vi "CRYMR_TOL2.vi"(0 "Tolerance":u16(ring)=1 items=["Individual Points", "Absolute Limits", "Floating Limits", "Floating Data", "Aligned Limits", "Aligned Data"], 1 "X Floating Limits":u16(ring) items=["No", "Yes"], 2 "x axis":enum32{"Linear", "Log"}(ring), 5 "Limits":u16(ring)=2 items=["Upper Only", "Lower Only", "Upper & Lower"], 6 "X min-max-step":T1={"Limit X Offset Min"=0.0, "Limit X Offset Max"=500.0, "Limit X Offset Step Size"=10.0} {"Limit X Offset Step Size" step=0.01 format="%.2f"; "Limit X Offset Max" step=0.01 format="%.2f"; "Limit X Offset Min" step=0.01 format="%.2f"}, 7 "Data":cluster{"Hz":dbl, "dB":dbl}[](array[cluster])=[{"Hz"=200.0, "dB"=2.9}, {"Hz"=500.0, "dB"=3.5}, {"Hz"=1000.0, "dB"=5.0}, {"Hz"=2000.0, "dB"=6.0}, {"Hz"=4500.0, "dB"=4.0}] {"dB" format="%.1f"}, 9 "Upper Limit":cluster{"Hz":dbl, "y":dbl}[](array[cluster])=[{"Hz"=300.0, "y"=4.0}, {"Hz"=1000.0, "y"=6.5}, {"Hz"=4000.0, "y"=5.0}, {"Hz"=5000.0, "y"=4.2}] {"y" format="%.1f"}, 11 "Lower Limit":cluster{"Hz":dbl, "y":dbl}[](array[cluster])=[{"Hz"=400.0, "y"=0.5}, {"Hz"=1000.0, "y"=3.5}, {"Hz"=3000.0, "y"=1.5}] {"y" format="%.1f"}, 12 "Align Reference":cluster{dbl, dbl}={1250.0, 4.5} {"?" format="%.1f"}, 13 "Resolution (decimals)":i32=2) -> (3 "Margin":dbl=-0.25 format="%.1f", 4 "Verdict":bool, 8 "Data Out":cluster{dbl, dbl}[](array[cluster])=[{200.00000000000003, 2.9}, {499.99999999999994, 3.5}, {1000.0, 5.0}, {2000.0000000000002, 6.0}, {4499.999999999998, 4.0}] {"?" format="%.2f"; "?" format="%.2f"}, 10 "Upper Limit Out":cluster{dbl, dbl}[](array[cluster])=[{300.0000000000001, 4.0}, {1000.0, 6.5}, {4000.000000000001, 5.0}, {4999.999999999999, 4.2}] {"?" format="%.2f"; "?" format="%.2f"}, 14 "Align Reference Out":cluster{dbl, dbl}={1250.0, 4.5} {"?" format="%.1f"}, 15 "Lower Limit Out":cluster{dbl, dbl}[](array[cluster])=[{400.0000000000001, 0.5}, {1000.0, 3.5}, {3000.000000000001, 1.5}] {"?" format="%.2f"; "?" format="%.2f"})   [LabVIEW 2013]
uses:
  CRYLimit edit global.vi
panel:
  out "Lo Fail":cluster{dbl, dbl}[](array[cluster])
  out "Up Fail":cluster{dbl, dbl}[](array[cluster])
  out "verdict out":bool
  out "align ref point":cluster{dbl, dbl}[](array[cluster])
  out "Align Ref":cluster{dbl, dbl}
  out "Critical":cluster{dbl, dbl}[](array[cluster])
  out "Margin out":dbl
  out "Data output":cluster{dbl, dbl}[](array[cluster])
  out "Low out":cluster{dbl, dbl}[](array[cluster])
  out "Up out":cluster{dbl, dbl}[](array[cluster])
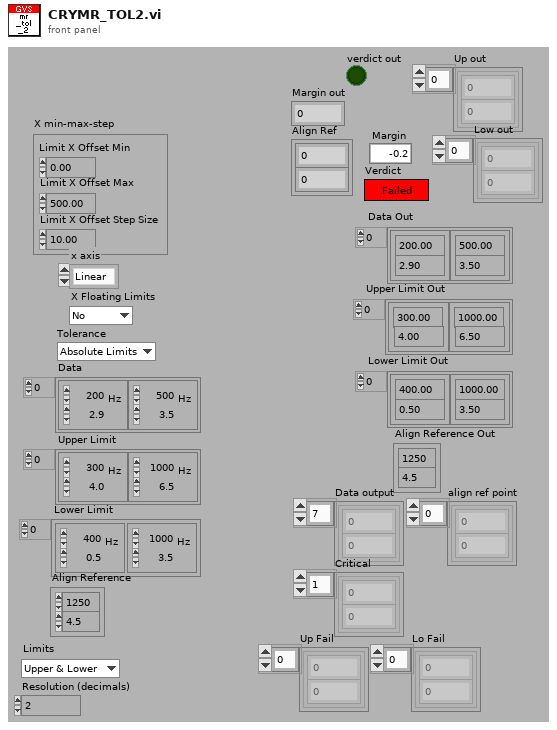
[diagram p1: front panel]
types:
  T1 = cluster{"Limit X Offset Min":dbl, "Limit X Offset Max":dbl, "Limit X Offset Step Size":dbl}
  T2 = cluster{"Data X Offset":dbl, "Data Y Offset":dbl}
  T3 = cluster{"Limit X Offset Min":dbl, "Limit Y Offset":dbl}
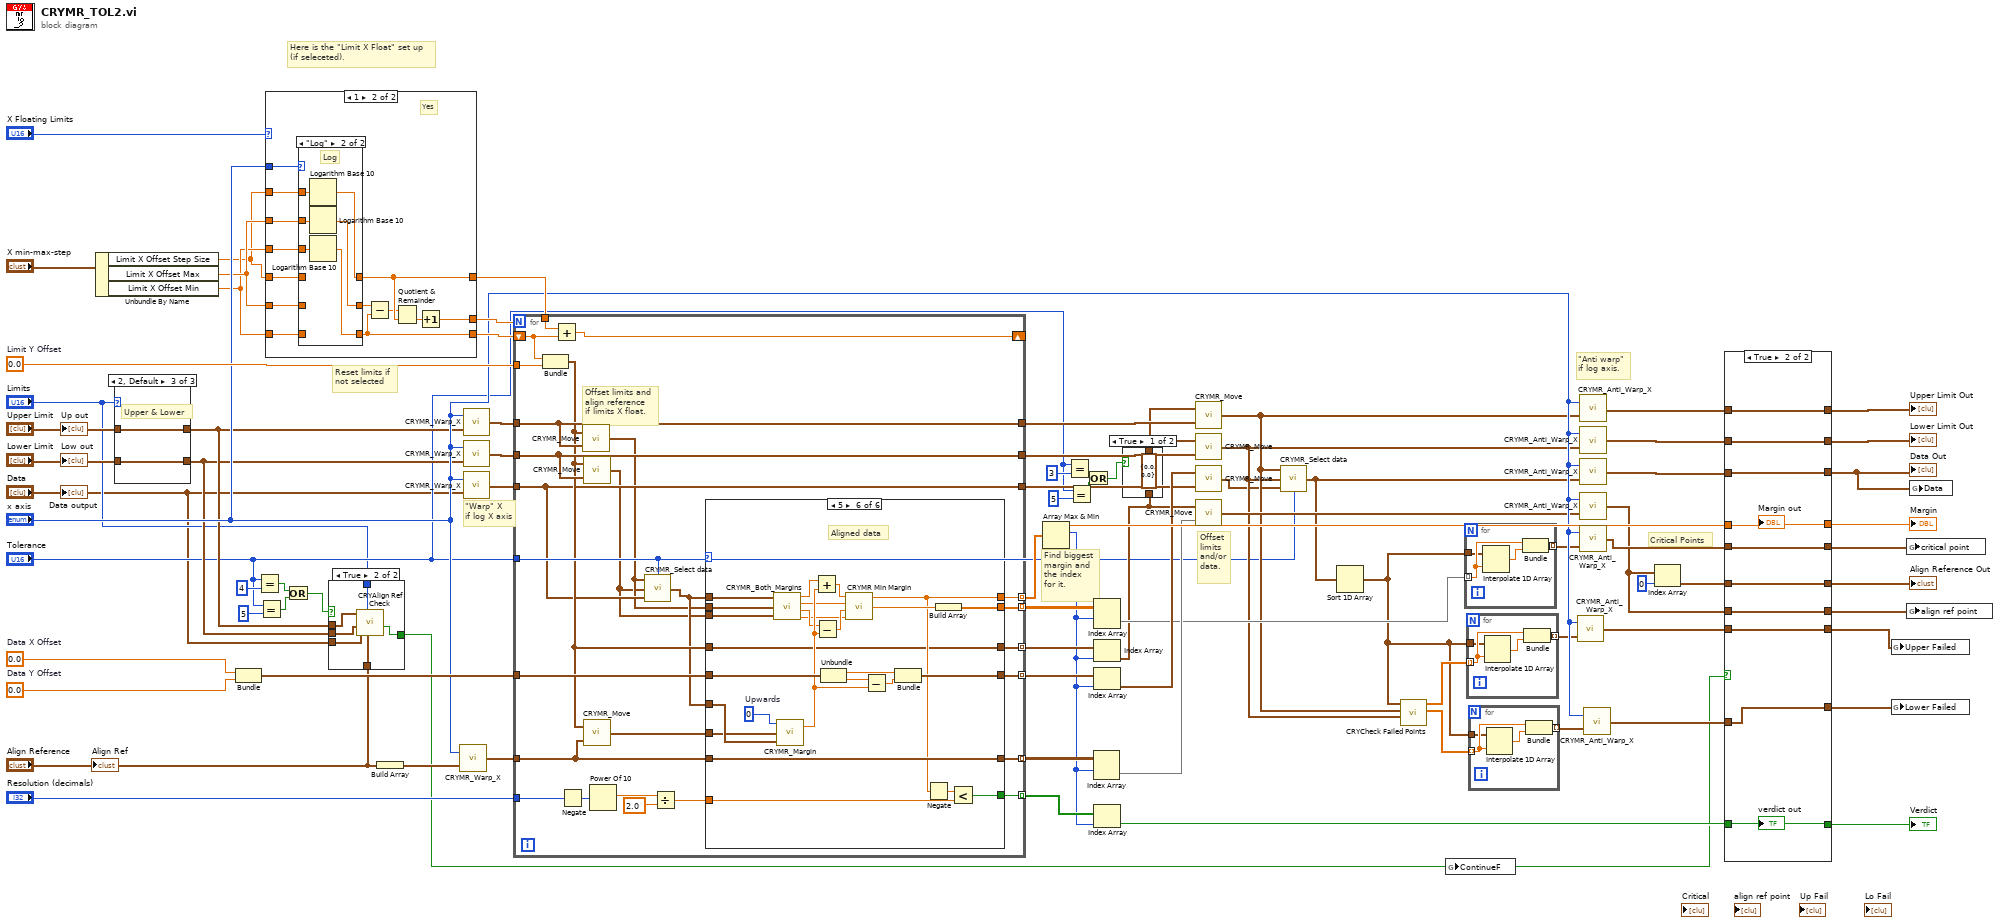
[diagram p0: block diagram]
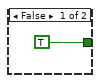
[diagram p3: hidden frame]
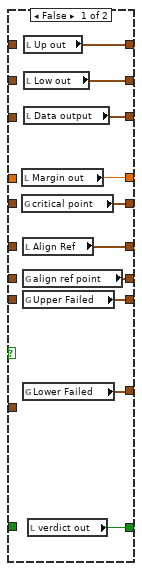
[diagram p4: hidden frame]
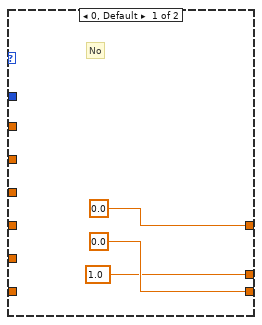
[diagram p5: hidden frame]
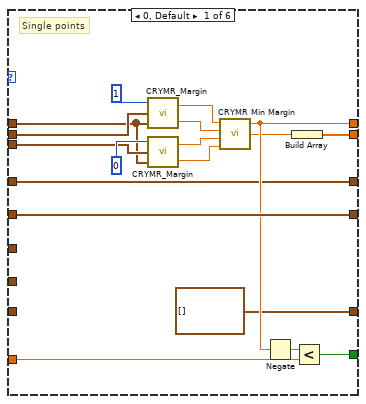
[diagram p7: hidden frame]
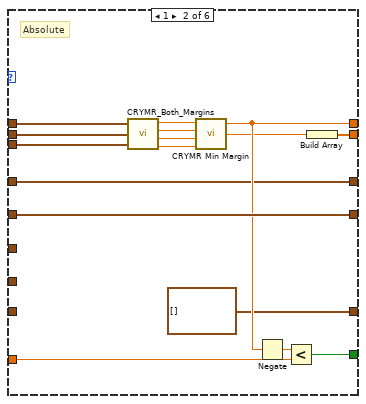
[diagram p8: hidden frame]
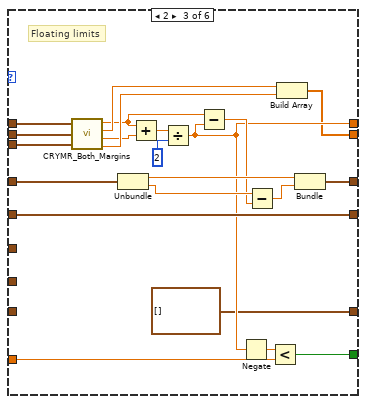
[diagram p9: hidden frame]
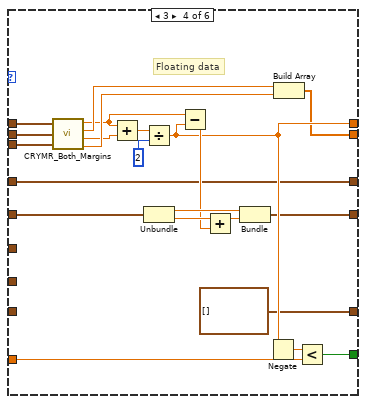
[diagram p10: hidden frame]
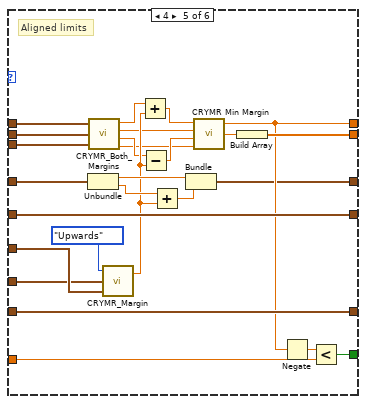
[diagram p11: hidden frame]
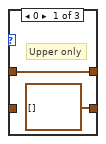
[diagram p12: hidden frame]
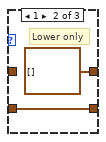
[diagram p13: hidden frame]
diagram:
  w56 = 0.0  # Data Y Offset
  w57 = 0.0  # Data X Offset
  w61 = 0.0  # Limit Y Offset
  # "\"Anti warp\"\nif log axis."
  # "Critical Points"
  # "Find biggest\nmargin and \nthe index\nfor it."
  # "Offset \nlimits\nand/or\ndata."
  # "\"Warp\" X \nif log X axis"
  # "Reset limits if \nnot selected"
  # "Here is the \"Limit X Float\" set up\n(if seleceted)."
  n1 = Unbundle By Name("X min-max-step") -> ("Limit X Offset Step Size"=w38:dbl, "Limit X Offset Max"=w40:dbl, "Limit X Offset Min"=w39:dbl)
  n2 = case shown="2, Default" "Limits" {
    tunnel: "Upper Limit" -> [w87 _ w91]
    tunnel: [w87 cluster{"Hz":dbl, "y":dbl}[] [] ("Upper Limit") w91] -> w29
    tunnel: "Lower Limit" -> [_ w89 w90]
    tunnel: [cluster{"Hz":dbl, "y":dbl}[] [] ("Lower Limit") w89 w90] -> w28
    frame 0 {
      # "Upper only"
    }
    frame 1 {
      # "Lower only"
    }
    frame 2, Default {
      # "Upper & Lower"
    }
  }
  n3 = Bundle("Data X Offset"=w57, "Data Y Offset"=w56) -> (w52:T2)  [unwired: 1 out]
  n4 = Equal?(x="Tolerance", y=u16 4) -> (x = y?=w17:bool)
  n5 = Equal?(x="Tolerance", y=u16 5) -> (x = y?=w16:bool)
  n6 = case shown="1" "X Floating Limits" {
    tunnel: w38 -> [_ w101]
    tunnel: w40 -> [_ w103]
    tunnel: w39 -> [_ w106]
    tunnel: w39 -> [_ w104]
    tunnel: [0.0 w102] -> w43
    tunnel: w40 -> [_ w105]
    tunnel: [0.0 w100] -> w45
    tunnel: [1.0 w98] -> w44
    tunnel: "x axis" -> [_ w107]
    tunnel: w38 -> [_ w99]
    frame 0, Default {
      # "No"
    }
    frame 1 {
      # "Yes"
      n7 = case shown="\"Log\"" w107 {
        tunnel: w106 -> [_ w116]
        tunnel: w105 -> [w110 _]
        tunnel: [w110 w113] -> w97
        tunnel: w104 -> [w109 _]
        tunnel: [w109 w114] -> w102
        tunnel: w103 -> [_ w115]
        tunnel: w101 -> [w108 _]
        tunnel: [w108 w111] -> w100
        tunnel: w99 -> [_ w112]
        frame "Linear", Default {
          # "Lin"
        }
        frame "Log" {
          # "Log"
          n8 = Logarithm Base 10(1:w112) -> (0:w111:dbl)
          n9 = Logarithm Base 10(1:w115) -> (0:w113:dbl)
          n10 = Logarithm Base 10(1:w116) -> (0:w114:dbl)
        }
      }
      n11 = Subtract(x=w97, y=w102) -> (x-y=w96:dbl)
      n12 = Quotient & Remainder(x=w96, y=w100) -> (floor(x/y)=w95:dbl)  [unwired: 1 out]
      n13 = Increment(x=w95) -> (x+1=w98:dbl)
    }
  }
  n14 = Or(x=w17, y=w16) -> (x .or. y?=w3:bool)
  n15 = case shown="True" w3 {
    tunnel: w29 -> [_ w123]
    tunnel: w28 -> [_ w122]
    tunnel: "Align Reference" -> [_ w121]
    tunnel: [TRUE ("Align Flag") w118] -> w12
    tunnel: "Limits" -> [_ w120]
    tunnel: "Data" -> [_ w119]
    frame False {
    }
    frame True {
      n16 = call "CRYAlign Ref Check.vi"("Align Reference"=w121, "Limits"=w120, "Data"=w119, "Lower Limit"=w122, "Upper Limit"=w123) -> ("Align Flag"=w118:bool)  [unwired: 6 in]
    }
  }
  n17 = Build Array("Align Reference") -> (w51:cluster{dbl, dbl}[])
  n18 = call "CRYMR_Warp_X.vi"("Input"=w51, "x axis"="x axis") -> ("Output"=w50:cluster{dbl, dbl}[])
  n19 = call "CRYMR_Warp_X.vi"("Input"=w29, "x axis"="x axis") -> ("Output"=w53:cluster{dbl, dbl}[])
  n20 = call "CRYMR_Warp_X.vi"("Input"=w28, "x axis"="x axis") -> ("Output"=w54:cluster{dbl, dbl}[])
  n21 = call "CRYMR_Warp_X.vi"("Input"="Data", "x axis"="x axis") -> ("Output"=w49:cluster{dbl, dbl}[])
  n22 = for {
    N: w44 -> [_]
    tunnel: "Resolution (decimals)" -> [w129]
    tunnel: "Tolerance" -> [w124]
    tunnel: w54 -> [w134]
    tunnel: w53 -> [w135]
    tunnel: [w128] -> w64
    tunnel: [w134] -> w63
    tunnel: [w135] -> w62
    tunnel: [w144] -> w47 mode=indexing
    tunnel: [w143] -> w66 mode=indexing
    tunnel: [w142] -> w67 mode=indexing
    tunnel: [w141] -> w68 mode=indexing
    tunnel: w61 -> [w131]
    tunnel: [w140] -> w60 mode=indexing
    tunnel: w50 -> [w133]
    shift-right: [w138] -> _
    shift-left: w43 -> [w132]
    tunnel: [w137] -> w58 mode=indexing
    tunnel: w49 -> [w128]
    tunnel: w45 -> [w136]
    tunnel: w52 -> [w145]
    # "Offset limits and\nalign reference\nif limits X float."
    n23 = Bundle("Limit X Offset Min"=w132, "Limit Y Offset"=w131) -> (w130:T3)  [unwired: 1 out]
    n24 = Add(x=w136, y=w132) -> (x+y=w138:dbl)
    n25 = Negate(x=w129) -> (-x=w147:i32)
    n26 = call "CRYMR_Move.vi"("Input"=w135, "Offsets"=w130) -> ("Output"=w126:cluster{dbl, dbl}[])
    n27 = call "CRYMR_Move.vi"("Input"=w134, "Offsets"=w130) -> ("Output"=w125:cluster{dbl, dbl}[])
    n28 = call "CRYMR_Move.vi"("Input"=w133, "Offsets"=w130) -> ("Output"=w139:cluster{dbl, dbl}[])
    n29 = Power Of 10(x=w147) -> (10^x=w146:dbl)
    n30 = call "CRYMR_Select data.vi"("Tolerance"=w124, "Data"=w128, "Lower Limit"=w125, "Upper Limit"=w126) -> ("Data Out"=w127:cluster{dbl, dbl}[])
    n31 = Divide(x=w146, y=2.0) -> (x/y=w149:dbl)
    n32 = case shown="5" w124 {
      tunnel: [w166 w182 w201 w223 w252 w277] -> w141
      tunnel: w149 -> [w165 w181 w202 w224 w253 w278]
      tunnel: w127 -> [w150 w168 w186 w208 w244 w257]
      tunnel: w126 -> [w156 w170 w185 w207 w243 w256]
      tunnel: w125 -> [w155 w169 w184 w206 w242 w255]
      tunnel: w145 -> [w164 w180 w200 w209 w251 w269]
      tunnel: [w164 w180 w200 w217 w251 w268] -> w142
      tunnel: [w159 w172 w195 w210 w228 w254] -> w143
      tunnel: [w163 w179 w194 w218 w246 w258] -> w144
      tunnel: [w162 w177 w193 w216 w249 w265] -> w140
      tunnel: w127 -> [_ _ _ _ w250 w274]
      tunnel: w139 -> [_ _ _ _ w248 w264]
      tunnel: [cluster{dbl, dbl}[] [] cluster{dbl, dbl}[] [] cluster{dbl, dbl}[] [] cluster{dbl, dbl}[] [] w247 w263] -> w137
      tunnel: w133 -> [_ _ _ _ w247 w263]
      tunnel: w130 -> [w159 w172 w187 w210 w245 w254]
      frame 0, Default {
        # "Single points"
        n33 = call "CRYMR_Margin.vi"("To"=w150, "From"=w156, "Direction"=1) -> ("X"=w153:dbl, "Margin"=w154:dbl)
        n34 = call "CRYMR_Margin.vi"("To"=w150, "From"=w155, "Direction"=0) -> ("X"=w151:dbl, "Margin"=w152:dbl)
        n35 = call "CRYMR Min Margin.vi"("Lower X"=w151, "Lower Margin"=w152, "Upper X"=w153, "Upper Margin"=w154) -> ("X"=w161:dbl, "Min Margin"=w163:dbl)  [unwired: 1 out]
        n36 = Negate(x=w163) -> (-x=w167:dbl)
        n37 = Build Array(w161) -> (w162:dbl[])
        n38 = Less?(x=w167, y=w165) -> (x < y?=w166:bool)
      }
      frame 1 {
        # "Absolute"
        n39 = call "CRYMR_Both_Margins.vi"("Data"=w168, "Upper Limit"=w170, "Lower Limit"=w169) -> ("Upper Margin"=w171:dbl, "Upper Margin X"=w173:dbl, "Lower Margin"=w174:dbl, "Lower Margin X"=w175:dbl)
        n40 = call "CRYMR Min Margin.vi"("Lower X"=w175, "Lower Margin"=w174, "Upper X"=w173, "Upper Margin"=w171) -> ("X"=w178:dbl, "Min Margin"=w179:dbl)  [unwired: 1 out]
        n41 = Negate(x=w179) -> (-x=w183:dbl)
        n42 = Less?(x=w183, y=w181) -> (x < y?=w182:bool)
        n43 = Build Array(w178) -> (w177:dbl[])
      }
      frame 2 {
        # "Floating limits"
        n44 = call "CRYMR_Both_Margins.vi"("Data"=w186, "Upper Limit"=w185, "Lower Limit"=w184) -> ("Upper Margin"=w189:dbl, "Upper Margin X"=w190:dbl, "Lower Margin"=w188:dbl, "Lower Margin X"=w191:dbl)
        n45 = Unbundle(w187) -> ("Limit X Offset Min"=w199:dbl, "Limit Y Offset"=w198:dbl)
        n46 = Add(x=w189, y=w188) -> (x+y=w205:dbl)
        n47 = Divide(x=w205, y=2) -> (x/y=w194:dbl)
        n48 = Subtract(x=w189, y=w194) -> (x-y=w196:dbl)
        n49 = Negate(x=w194) -> (-x=w203:dbl)
        n50 = Subtract(x=w198, y=w196) -> (x-y=w197:dbl)
        n51 = Less?(x=w203, y=w202) -> (x < y?=w201:bool)
        n52 = Build Array(w190, w191) -> (w193:dbl[])
        n53 = Bundle("Limit X Offset Min"=w199, w197) -> (w195:cluster{"Limit X Offset Min":dbl, dbl})  [unwired: 1 out]
      }
      frame 3 {
        # "Floating data"
        n54 = call "CRYMR_Both_Margins.vi"("Data"=w208, "Upper Limit"=w207, "Lower Limit"=w206) -> ("Upper Margin"=w212:dbl, "Upper Margin X"=w213:dbl, "Lower Margin"=w211:dbl, "Lower Margin X"=w214:dbl)
        n55 = Add(x=w212, y=w211) -> (x+y=w227:dbl)
        n56 = Divide(x=w227, y=2) -> (x/y=w218:dbl)
        n57 = Unbundle(w209) -> ("Data X Offset"=w222:dbl, "Data Y Offset"=w221:dbl)
        n58 = Subtract(x=w212, y=w218) -> (x-y=w219:dbl)
        n59 = Add(x=w221, y=w219) -> (x+y=w220:dbl)
        n60 = Bundle("Data X Offset"=w222, w220) -> (w217:cluster{"Data X Offset":dbl, dbl})  [unwired: 1 out]
        n61 = Negate(x=w218) -> (-x=w225:dbl)
        n62 = Build Array(w213, w214) -> (w216:dbl[])
        n63 = Less?(x=w225, y=w224) -> (x < y?=w223:bool)
      }
      frame 4 {
        # "Aligned limits"
        n64 = Unbundle(w245) -> ("Limit X Offset Min"=w240:dbl, "Limit Y Offset"=w239:dbl)
        n65 = call "CRYMR_Both_Margins.vi"("Data"=w244, "Upper Limit"=w243, "Lower Limit"=w242) -> ("Upper Margin"=w233:dbl, "Upper Margin X"=w232:dbl, "Lower Margin"=w231:dbl, "Lower Margin X"=w230:dbl)
        n66 = call "CRYMR_Margin.vi"("To"=w250, "From"=w248, "Direction"=enum16{"Upwards", "Downwards"}."Upwards") -> ("Margin"=w235:dbl)  [unwired: 1 out]
        n67 = Add(x=w233, y=w235) -> (x+y=w237:dbl)
        n68 = Subtract(x=w231, y=w235) -> (x-y=w236:dbl)
        n69 = Add(x=w239, y=w235) -> (x+y=w238:dbl)
        n70 = Bundle("Limit X Offset Min"=w240, w238) -> (w228:cluster{"Limit X Offset Min":dbl, dbl})  [unwired: 1 out]
        n71 = call "CRYMR Min Margin.vi"("Lower X"=w230, "Lower Margin"=w236, "Upper X"=w232, "Upper Margin"=w237) -> ("X"=w234:dbl, "Min Margin"=w246:dbl)  [unwired: 1 out]
        n72 = Build Array(w234) -> (w249:dbl[])
        n73 = Negate(x=w246) -> (-x=w241:dbl)
        n74 = Less?(x=w241, y=w253) -> (x < y?=w252:bool)
      }
      frame 5 {
        w273 = 0  # Upwards
        # "Aligned data"
        n75 = call "CRYMR_Both_Margins.vi"("Data"=w257, "Upper Limit"=w256, "Lower Limit"=w255) -> ("Upper Margin"=w262:dbl, "Upper Margin X"=w260:dbl, "Lower Margin"=w261:dbl, "Lower Margin X"=w259:dbl)
        n76 = call "CRYMR_Margin.vi"("To"=w274, "From"=w264, "Direction"=w273) -> ("Margin"=w267:dbl)  [unwired: 1 out]
        n77 = Add(x=w262, y=w267) -> (x+y=w272:dbl)
        n78 = Subtract(x=w261, y=w267) -> (x-y=w271:dbl)
        n79 = Unbundle(w269) -> ("Data X Offset"=w276:dbl, "Data Y Offset"=w275:dbl)
        n80 = call "CRYMR Min Margin.vi"("Lower X"=w259, "Lower Margin"=w271, "Upper X"=w260, "Upper Margin"=w272) -> ("X"=w266:dbl, "Min Margin"=w258:dbl)  [unwired: 1 out]
        n81 = Subtract(x=w275, y=w267) -> (x-y=w270:dbl)
        n82 = Bundle("Data X Offset"=w276, w270) -> (w268:cluster{"Data X Offset":dbl, dbl})  [unwired: 1 out]
        n83 = Negate(x=w258) -> (-x=w279:dbl)
        n84 = Build Array(w266) -> (w265:dbl[])
        n85 = Less?(x=w279, y=w278) -> (x < y?=w277:bool)
      }
    }
  }
  n86 = Array Max & Min(array=w47) -> (max value=w84:dbl, max index (indices)=w46:i32)  [unwired: 2 out]
  n87 = Equal?(x="Tolerance", y=u16 3) -> (x = y?=w8:bool)
  n88 = Equal?(x="Tolerance", y=u16 5) -> (x = y?=w9:bool)
  n89 = Or(x=w8, y=w9) -> (x .or. y?=w5:bool)
  n90 = Index Array(array=w58, index (row)=w46) -> (element=w59:cluster{dbl, dbl}[])  [unwired: 1 in]
  n91 = Index Array(array=w60, index (row)=w46) -> (element=w55:dbl[])  [unwired: 1 in]
  n92 = Index Array(array=w66, index=w46) -> (element=w11:T3)
  n93 = Index Array(array=w67, index=w46) -> (element=w65:T2)
  n94 = Index Array(array=w68, index=w46) -> (element=w85:bool)
  n95 = case shown="True" w5 {
    tunnel: w11 -> [_ w281]
    tunnel: [T3 {"Limit X Offset Min"=0.0, "Limit Y Offset"=0.0} w281] -> w10
    frame True {
    }
    frame False {
    }
  }
  n96 = call "CRYMR_Move.vi"("Input"=w62, "Offsets"=w10) -> ("Output"=w27:cluster{dbl, dbl}[])
  n97 = call "CRYMR_Move.vi"("Input"=w63, "Offsets"=w10) -> ("Output"=w26:cluster{dbl, dbl}[])
  n98 = call "CRYMR_Move.vi"("Input"=w64, "Offsets"=w65) -> ("Output"=w25:cluster{dbl, dbl}[])
  n99 = call "CRYMR_Move.vi"("Input"=w59, "Offsets"=w11) -> ("Output"=w37:cluster{dbl, dbl}[])
  n100 = call "CRYMR_Select data.vi"("Tolerance"="Tolerance", "Data"=w25, "Lower Limit"=w26, "Upper Limit"=w27) -> ("Data Out"=w24:cluster{dbl, dbl}[])
  n101 = Sort 1D Array(array=w24) -> (sorted array=w30:cluster{dbl, dbl}[])
  n102 = call "CRYCheck Failed Points.vi"("Low Limit"=w26, "Up Limit"=w27, "Data"=w30) -> ("Low Failed_X"=w31:dbl[], "Up Failed_X"=w32:dbl[])  [unwired: 7 out]
  n103 = global write "CRYLimit edit global.vi" "ContinueF"(w12) -> ()
  n104 = for {
    tunnel: w55 -> [w284] mode=indexing
    tunnel: w30 -> [w282]
    tunnel: [w283] -> w36 mode=indexing
    n105 = Interpolate 1D Array(1:w284, 2:w282) -> (0:w285:dbl)
    n106 = Bundle("X"=w284, w285) -> (w283:cluster{"X":dbl, dbl})  [unwired: 1 out]
  }
  n107 = for {
    tunnel: w32 -> [w288] mode=indexing
    tunnel: w30 -> [w286]
    tunnel: [w287] -> w34 mode=indexing
    n108 = Interpolate 1D Array(1:w288, 2:w286) -> (0:w289:dbl)
    n109 = Bundle(w288, w289) -> (w287:cluster{dbl, dbl})  [unwired: 1 out]
  }
  n110 = for {
    tunnel: w31 -> [w292] mode=indexing
    tunnel: w30 -> [w290]
    tunnel: [w291] -> w33 mode=indexing
    n111 = Interpolate 1D Array(1:w292, 2:w290) -> (0:w293:dbl)
    n112 = Bundle(w292, w293) -> (w291:cluster{dbl, dbl})  [unwired: 1 out]
  }
  n113 = call "CRYMR_Anti_Warp_X.vi"("Input"=w34, "x axis"="x axis") -> ("Output"=w23:cluster{dbl, dbl}[])
  n114 = call "CRYMR_Anti_Warp_X.vi"("Input"=w27, "x axis"="x axis") -> ("Output"=w83:cluster{dbl, dbl}[])
  n115 = call "CRYMR_Anti_Warp_X.vi"("Input"=w26, "x axis"="x axis") -> ("Output"=w82:cluster{dbl, dbl}[])
  n116 = call "CRYMR_Anti_Warp_X.vi"("Input"=w24, "x axis"="x axis") -> ("Output"=w81:cluster{dbl, dbl}[])
  n117 = call "CRYMR_Anti_Warp_X.vi"("Input"=w37, "x axis"="x axis") -> ("Output"=w78:cluster{dbl, dbl}[])
  n118 = call "CRYMR_Anti_Warp_X.vi"("Input"=w36, "x axis"="x axis") -> ("Output"=w79:cluster{dbl, dbl}[])
  n119 = call "CRYMR_Anti_Warp_X.vi"("Input"=w33, "x axis"="x axis") -> ("Output"=w22:cluster{dbl, dbl}[])
  n120 = Index Array(array=w78, index=0 ("Index")) -> (element=w80:cluster{dbl, dbl})
  n121 = case shown="True" w12 {
    tunnel: w83 -> [_ w312]
    tunnel: w82 -> [_ w311]
    tunnel: w81 -> [_ w310]
    tunnel: w84 -> [_ w313]
    tunnel: w80 -> [_ w309]
    tunnel: w85 -> [_ w306]
    tunnel: w79 -> [_ w308]
    tunnel: w78 -> [_ w307]
    tunnel: [w303 w313] -> w77
    tunnel: [w302 w312] -> w76
    tunnel: [w301 w311] -> w75
    tunnel: [w300 w310] -> w73
    tunnel: [w295 w309] -> w74
    tunnel: [w298 w308] -> w72
    tunnel: [w294 w307] -> w71
    tunnel: [w299 w306] -> w70
    tunnel: w23 -> [_ w305]
    tunnel: w22 -> [_ w304]
    tunnel: [w297 w305] -> w21
    tunnel: [w296 w304] -> w20
    frame False {
      n122 = local read "Margin out"() -> (w303:dbl)
      n123 = global read "CRYLimit edit global.vi" "critical point"() -> (w298:cluster{dbl, dbl}[])
      n124 = local read "Align Ref"() -> (w295:cluster{dbl, dbl})
      n125 = global read "CRYLimit edit global.vi" "align ref point"() -> (w294:cluster{dbl, dbl}[])
      n126 = global read "CRYLimit edit global.vi" "Upper Failed"() -> (w297:cluster{dbl, dbl}[])
      n127 = global read "CRYLimit edit global.vi" "Lower Failed"() -> (w296:cluster{dbl, dbl}[])
      n128 = local read "Up out"() -> (w302:cluster{dbl, dbl}[])
      n129 = local read "Low out"() -> (w301:cluster{dbl, dbl}[])
      n130 = local read "Data output"() -> (w300:cluster{dbl, dbl}[])
      n131 = local read "verdict out"() -> (w299:bool)
    }
    frame True {
      "Margin out" <- w313
      "verdict out" <- w306
    }
  }
  "Verdict" <- w70
  "Align Reference Out" <- w74
  "Margin" <- w77
  "Data Out" <- w73
  "Lower Limit Out" <- w75
  "Upper Limit Out" <- w76
  n132 = global write "CRYLimit edit global.vi" "Upper Failed"(w21) -> ()
  n133 = global write "CRYLimit edit global.vi" "Lower Failed"(w20) -> ()
  n134 = global write "CRYLimit edit global.vi" "critical point"(w72) -> ()
  n135 = global write "CRYLimit edit global.vi" "align ref point"(w71) -> ()
  n136 = global write "CRYLimit edit global.vi" "Data"(w73) -> ()
  "Up out" <- "Upper Limit"
  "Low out" <- "Lower Limit"
  "Data output" <- "Data"
  "Align Ref" <- "Align Reference"
